vi "Extract Numbers with Match Pattern 1.vi"() -> ()   [LabVIEW 2020]
panel:
  out "Input String Length":i32
  out "Offset Past Match":i32[](array[numeric])
  out "Numeric":i32
  out "Extracted Number":dbl[](array[numeric])
  in  "String":string="one 2 -3 4.0 5.5"
  # "OverView :"
  # "Note :"
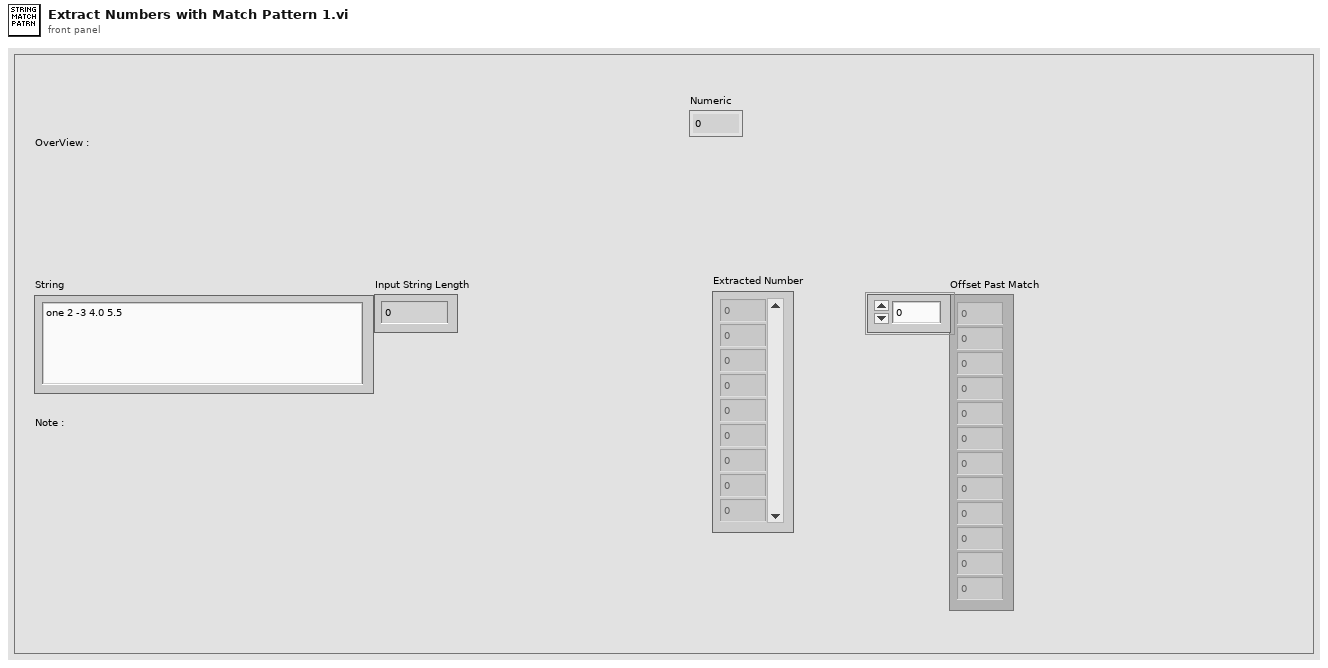
[diagram p1: front panel]
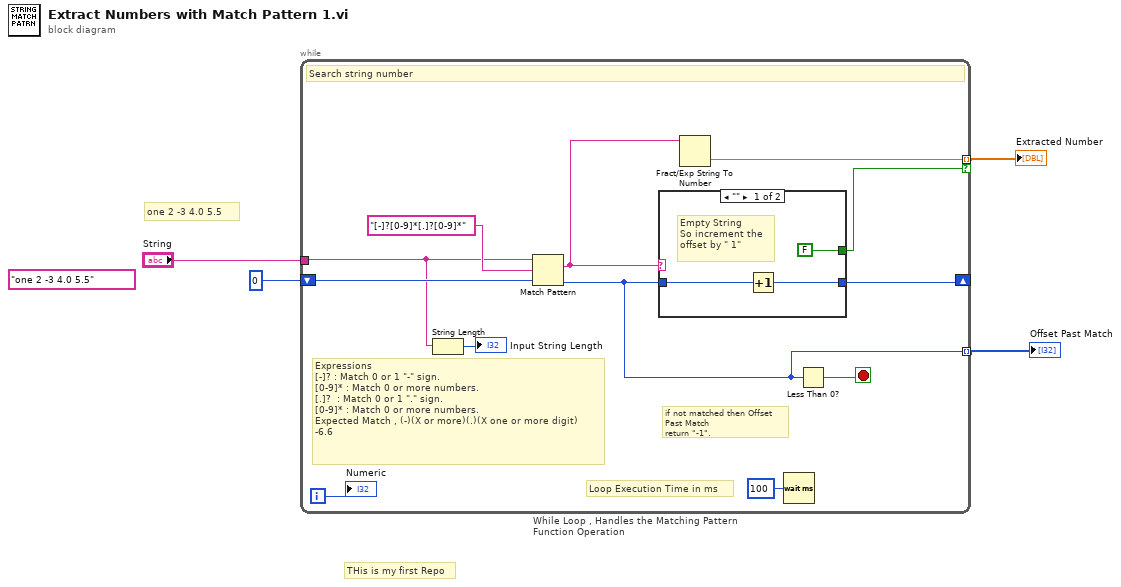
[diagram p0: block diagram]
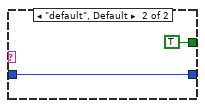
[diagram p2: hidden frame]
diagram:
  (unwired) "one 2 -3 4.0 5.5" ("String")
  # "THis is my first Repo"
  # "one 2 -3 4.0 5.5"
  n1 = while "While Loop , Handles the Matching Pattern Function Operation" {
    tunnel: "String" -> [w10]
    shift-right: [w11] -> _
    shift-left: 0 -> [w15]
    tunnel: [w14] -> w2 mode=indexing if=w7
    tunnel: [w5] -> w1 mode=indexing
    i -> [w12]
    stop <- w6 stop-if-true
    # "Expressions\n[-]? : Match 0 or 1 \"-\" sign.\n[0-9]* : Match 0 or more numbers.\n[.]?  : Match 0 or 1 \".\" sign.\n[0-9]* : Match 0 or more numbers.\nExpected Match , (-)(X or more)(.)(X one or more digit)\n-6.6"
    # "Loop Execution Time in ms"
    # "if not matched then Offset Past Match\nreturn \"-1\"."
    # "Search string number"
    n2 = String Length(string=w10) -> (length=→"Input String Length":i32)
    n3 = Match Pattern(string=w10, regular expression="[-]?[0-9]*[.]?[0-9]*", offset (0)=w15) -> (match substring=w8:string, offset past match=w5:i32)  [unwired: 2 out]
    n4 = case shown="\"\"" w8 {
      tunnel: w5 -> [w19 w21]
      tunnel: [w17 w21] -> w11
      tunnel: [FALSE TRUE] -> w7
      frame "" {
        # "Empty String \nSo increment the \noffset by \" 1\""
        n5 = Increment(x=w19) -> (x+1=w17:i32)
      }
      frame "default", Default {
      }
    }
    n6 = Fract/Exp String To Number(string=w8) -> (number=w14:dbl)  [unwired: 3 in, 1 out]
    n7 = Wait (ms)(milliseconds to wait=u32 100) -> ()  [unwired: 1 out]
    n8 = Less Than 0?(x=w5) -> (x < 0?=w6:bool)
    "Numeric" <- w12
  }
  "Extracted Number" <- w2
  "Offset Past Match" <- w1
